vi "ADC4Temp LaunchPad.vi"(11 "string":string) -> (1 "Temp (deg C)":dbl format="%#.1f", 2 "Temp (Volt)":dbl, 3 "ADCvalue":u16)   [LabVIEW 2011]
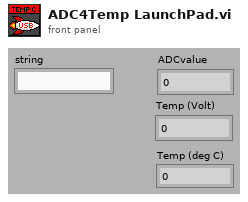
[diagram p1: front panel]
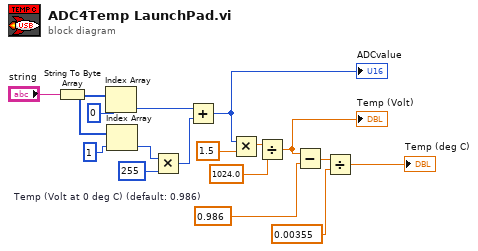
[diagram p0: block diagram]
diagram:
  w3 = 0.986  # Temp (Volt at 0 deg C) (default: 0.986)
  n1 = String To Byte Array(string="string") -> (unsigned byte array=w16:u8[])
  n2 = Index Array(array=w16, index=0) -> (element=w11:u8)
  n3 = Index Array(array=w16, index=1) -> (element=w14:u8)
  n4 = Multiply(x=w14, y=u16 255) -> (x*y=w12:u16)
  n5 = Add(x=w11, y=w12) -> (x+y=w10:u16)
  "ADCvalue" <- w10
  n6 = Multiply(x=w10, y=1.5) -> (x*y=w8:dbl)
  n7 = Divide(x=w8, y=1024.0) -> (x/y=w6:dbl)
  "Temp (Volt)" <- w6
  n8 = Subtract(x=w6, y=w3) -> (x-y=w5:dbl)
  n9 = Divide(x=w5, y=0.00355) -> (x/y=→"Temp (deg C)":dbl)
